vi "AH_ParseMSG.vi"(5 "InputMSG":string, 11 "error in (no error)":errorcluster) -> (4 "Cap":dbl, 6 "Los":dbl, 8 "ExVolt":dbl, 10 "Error":i32, 15 "error out":errorcluster)   [LabVIEW 2021]
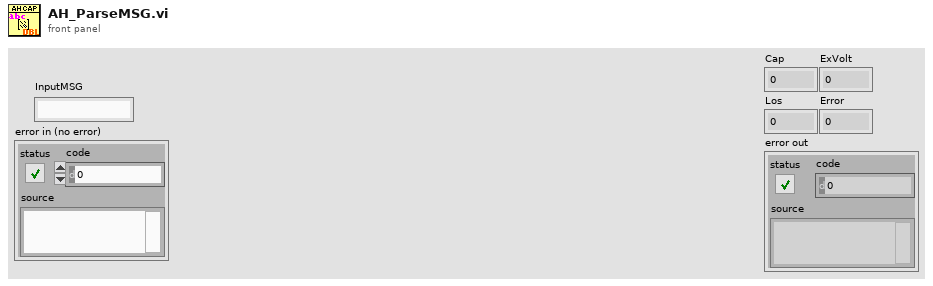
[diagram p1: front panel]
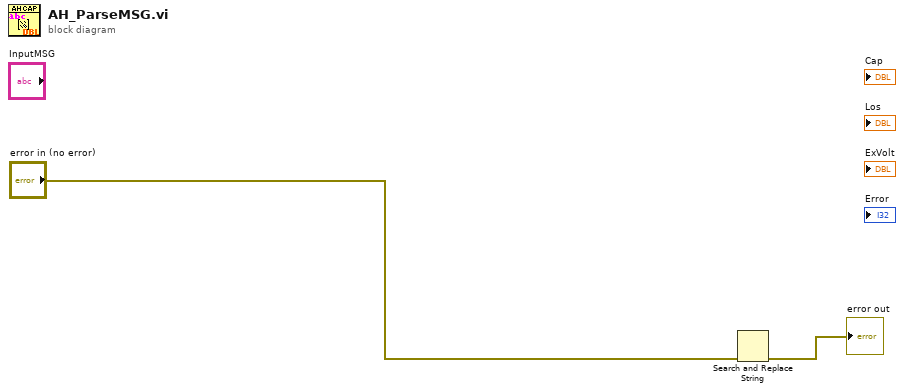
[diagram p0: block diagram]
diagram:
  n1 = Search and Replace String(error in="error in (no error)") -> (error out=→"error out":errorcluster)  [unwired: 7 in, 3 out]
